vi "ExecuteCommand.vi"(8 "error in":errorcluster, 9 "Command":string="whoami", 10 "Session Ref":refnum<k24>, 11 "Command Execution in":refnum<class "Command Execution.lvclass">) -> (0 "error out":errorcluster, 3 "Command Execution out":refnum<class "Command Execution.lvclass">)   [LabVIEW 2015, in "WinSCP.lvlib" / "Command Execution.lvclass"]
doc: "This method actually calls the WinSCP .NET API Method ExecuteCommand().\nThis method is synchronous and will actually only return when the command finishes executing on the distant target. Any blocking command should NOT be passed to this method since there is no way to abort a launched command."
uses:
  Command Execution.lvclass
  C:/Users/Public/Documents/Projects/lv-winscp/Bin WinSCP/WinSCPnet.dll
  Bin WinSCP/WinSCPnet.dll
  Command Execution.lvclass/Command Execution.ctl
  ErrorDescription.ctl
panel:
  out "Output":string
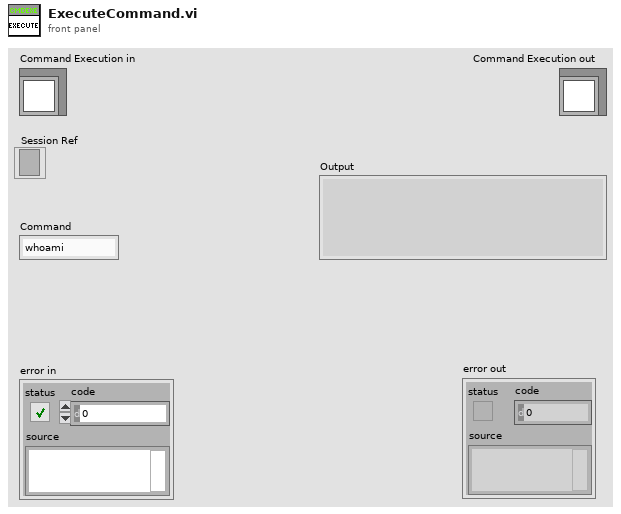
[diagram p1: front panel]
types:
  T1 = typedef "WinSCP.lvlib/Command Execution.lvclass/ErrorDescription.ctl" = cluster{"Message":string, "Source":string}
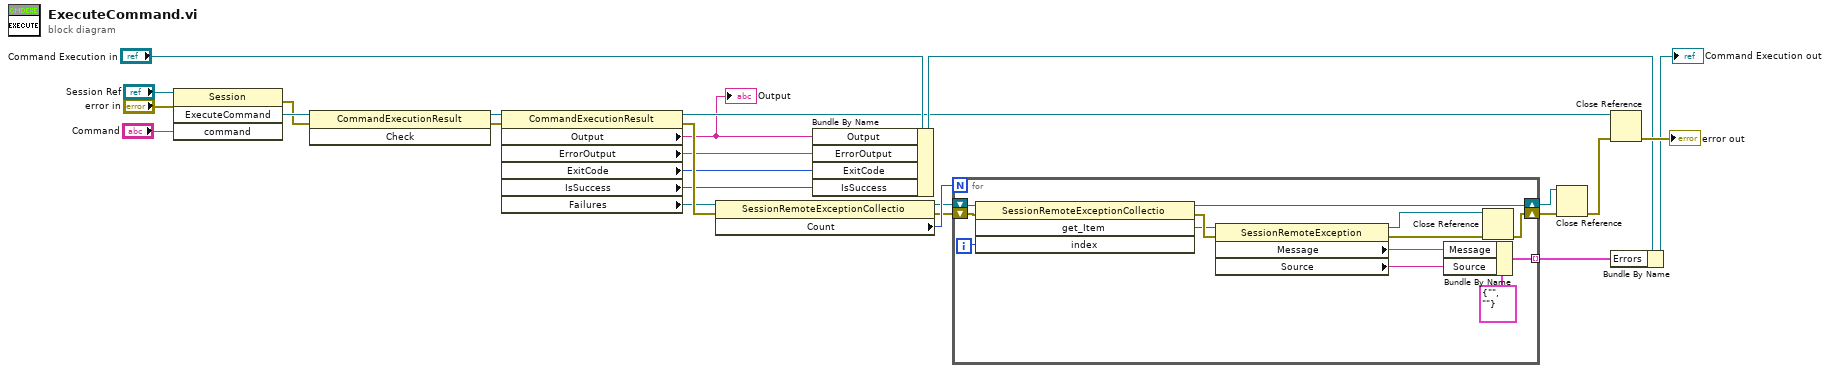
[diagram p0: block diagram]
diagram:
  n1 = invoke class="Session" method="ExecuteCommand"(reference="Session Ref", error in="error in", "command"="Command") -> (error out=w17:errorcluster, "ExecuteCommand"=w19:refnum<k24>)  [unwired: 1 in, 2 out]
  n2 = invoke class="CommandExecutionResult" method="Check"(reference=w19, error in=w17) -> (reference out=w20:refnum<k24>, error out=w16:errorcluster)  [unwired: 1 in, 1 out]
  n3 = property class="CommandExecutionResult"(reference=w20, error in=w16) -> (reference out=w15:refnum<k24>, error out=w21:errorcluster, "Output"=w1:string, "ErrorOutput"=w6:string, "ExitCode"=w5:i32, "IsSuccess"=w4:bool, "Failures"=w13:refnum<k24>)
  "Output" <- w1
  n4 = property class="SessionRemoteExceptionCollectio"(reference=w13, error in=w21) -> (reference out=w11:refnum<k24>, error out=w10:errorcluster, "Count"=w12:i32)
  n5 = Bundle By Name(cluster="Command Execution in", "Output"=w1, "ErrorOutput"=w6, "ExitCode"=w5, "IsSuccess"=w4) -> (w24:refnum<class "Command Execution.lvclass">)
  n6 = for {
    N: w12 -> [_]
    shift-right: [w35] -> w8
    shift-left: w11 -> [w38]
    shift-right: [w30] -> w9
    shift-left: w10 -> [w33]
    tunnel: [w26] -> w2 mode=indexing
    i -> [w37]
    n7 = invoke class="SessionRemoteExceptionCollectio" method="get_Item"(reference=w38, error in=w33, "index"=w37) -> (reference out=w35:refnum<k24>, error out=w36:errorcluster, "get_Item"=w34:refnum<k24>)  [unwired: 1 in, 1 out]
    n8 = property class="SessionRemoteException"(reference=w34, error in=w36) -> (reference out=w31:refnum<k24>, error out=w32:errorcluster, "Message"=w28:string, "Source"=w27:string)
    n9 = Bundle By Name(cluster=T1 {"Message"="", "Source"=""} ("Error"), "Message"=w28, "Source"=w27) -> (w26:T1)
    n10 = Close Reference(reference=w31, error in (no error)=w32) -> (error out=w30:errorcluster)
  }
  n11 = Close Reference(reference=w8, error in (no error)=w9) -> (error out=w7:errorcluster)
  n12 = Close Reference(reference=w15, error in (no error)=w7) -> (error out=→"error out":errorcluster)
  n13 = Bundle By Name(cluster=w24, "Errors"=w2) -> (→"Command Execution out":refnum<class "Command Execution.lvclass">)
